vi "Crop (Rectangle Size Greyscale).vi"(7 "Origin (Default: 0,0)":T2, 8 "error in (no error)":errorcluster, 9 "Cropped Size":T1, 10 "Greyscale Image Destination in":T3, 11 "Greyscale Image Source in":T3) -> (0 "error out":errorcluster, 1 "Computed Size":T1, 3 "Greyscale Image Destination":T3)   [LabVIEW 2020, in "image.lvlib"]
doc: "Crop the Source Image region specified by the top-left corner (origin) and the crop-size into the Destination Image."
uses:
  image.lvlib
  Greyscale Image.ctl
  common/Image Size (Integer).ctl
  common/Image Point (Integer).ctl
  2dc01dea-48f6-4df4-8727-934e95e7e307.vi
  <vilib>/Utility/error.llb/Error Cluster From Error Code.vi
  common/common.lvlib
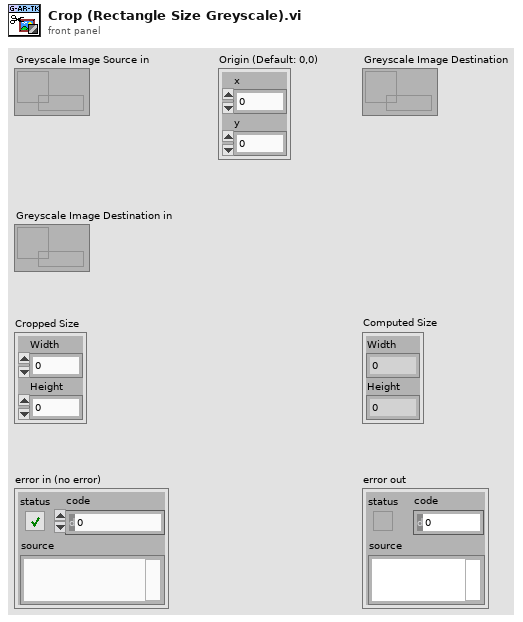
[diagram p1: front panel]
types:
  T1 = typedef "common.lvlib/Image Size (Integer).ctl" = cluster{"Width":u16, "Height":u16}
  T2 = typedef "common.lvlib/Image Point (Integer).ctl" = cluster{"x":i32, "y":i32}
  T3 = typedef "image.lvlib/Greyscale Image.ctl" = refnum<data-value>
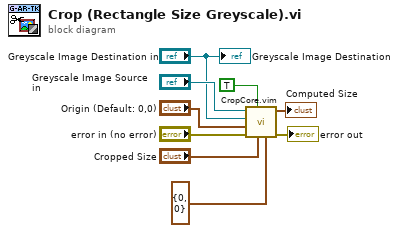
[diagram p0: block diagram]
diagram:
  n1 = call "CropCore.vim"("Other Point"=T2 {"x"=0, "y"=0}, "Size"="Cropped Size", "Use Size"=TRUE, "error in (no error)"="error in (no error)", "Origin"="Origin (Default: 0,0)", "Dst"="Greyscale Image Destination in", "Src"="Greyscale Image Source in") -> ("error out"=→"error out":errorcluster, "Computed Size"=→"Computed Size":T1)  [unwired: 3 in]
  "Greyscale Image Destination" <- "Greyscale Image Destination in"
